vi "Parameter XML Tx - Write old.vi"(0 "String (in)":string, 7 "Database []":T1) -> (4 "String (out)":string)   [LabVIEW 2017]
uses:
  <userlib>/_OpenG.lib/array/array.llb/Remove Duplicates from 1D Array (DBL)__ogtk.vi
  <userlib>/_OpenG.lib/array/array.llb/Filter 1D Array with Scalar (DBL)__ogtk.vi
  <userlib>/_OpenG.lib/array/array.llb/Index 1D Array Elements (DBL)__ogtk.vi
  Controls/Database_Array.ctl
  Controls/Encoding.ctl
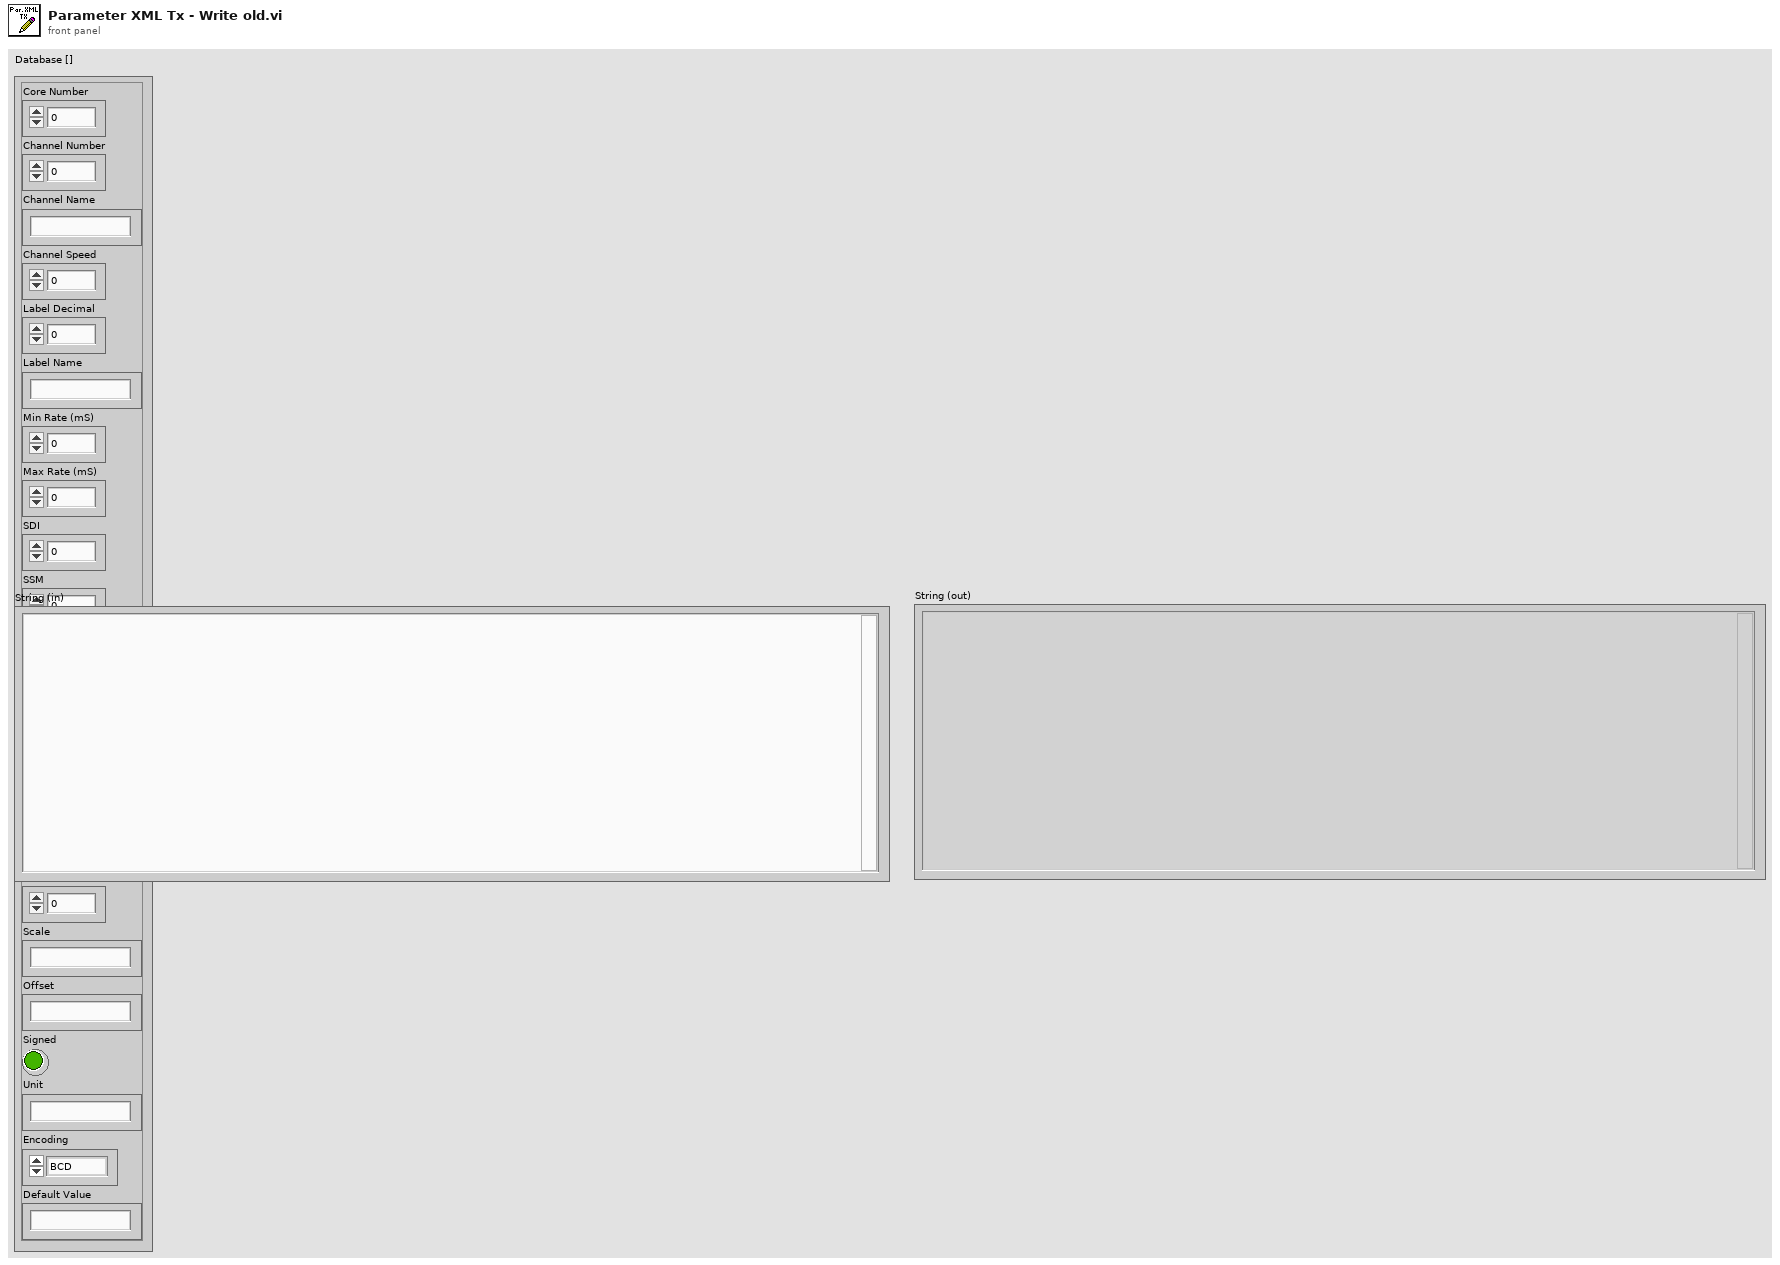
[diagram p1: front panel]
types:
  T1 = typedef "Database_Array.ctl" = cluster{"Core Number":i32, "Channel Number":i32, "Channel Name":string, "Channel Speed":i32, "Label Decimal":i32, "Label Name":string, "Min Rate (mS)":i32, "Max Rate (mS)":i32, "SDI":i32, "SSM":i32, "Create SDI":bool, "Create SSM":bool, "Create Parity":bool, "Parameter Name":string, "Start Bit":i32, "Number of Bits":i32, "Scale":string, "Offset":string, "Signed":bool, "Unit":string, "Encoding":T2, "Default Value":string}
  T2 = typedef "Encoding.ctl" = enum16{"BCD", "BNR", "Discrete"}
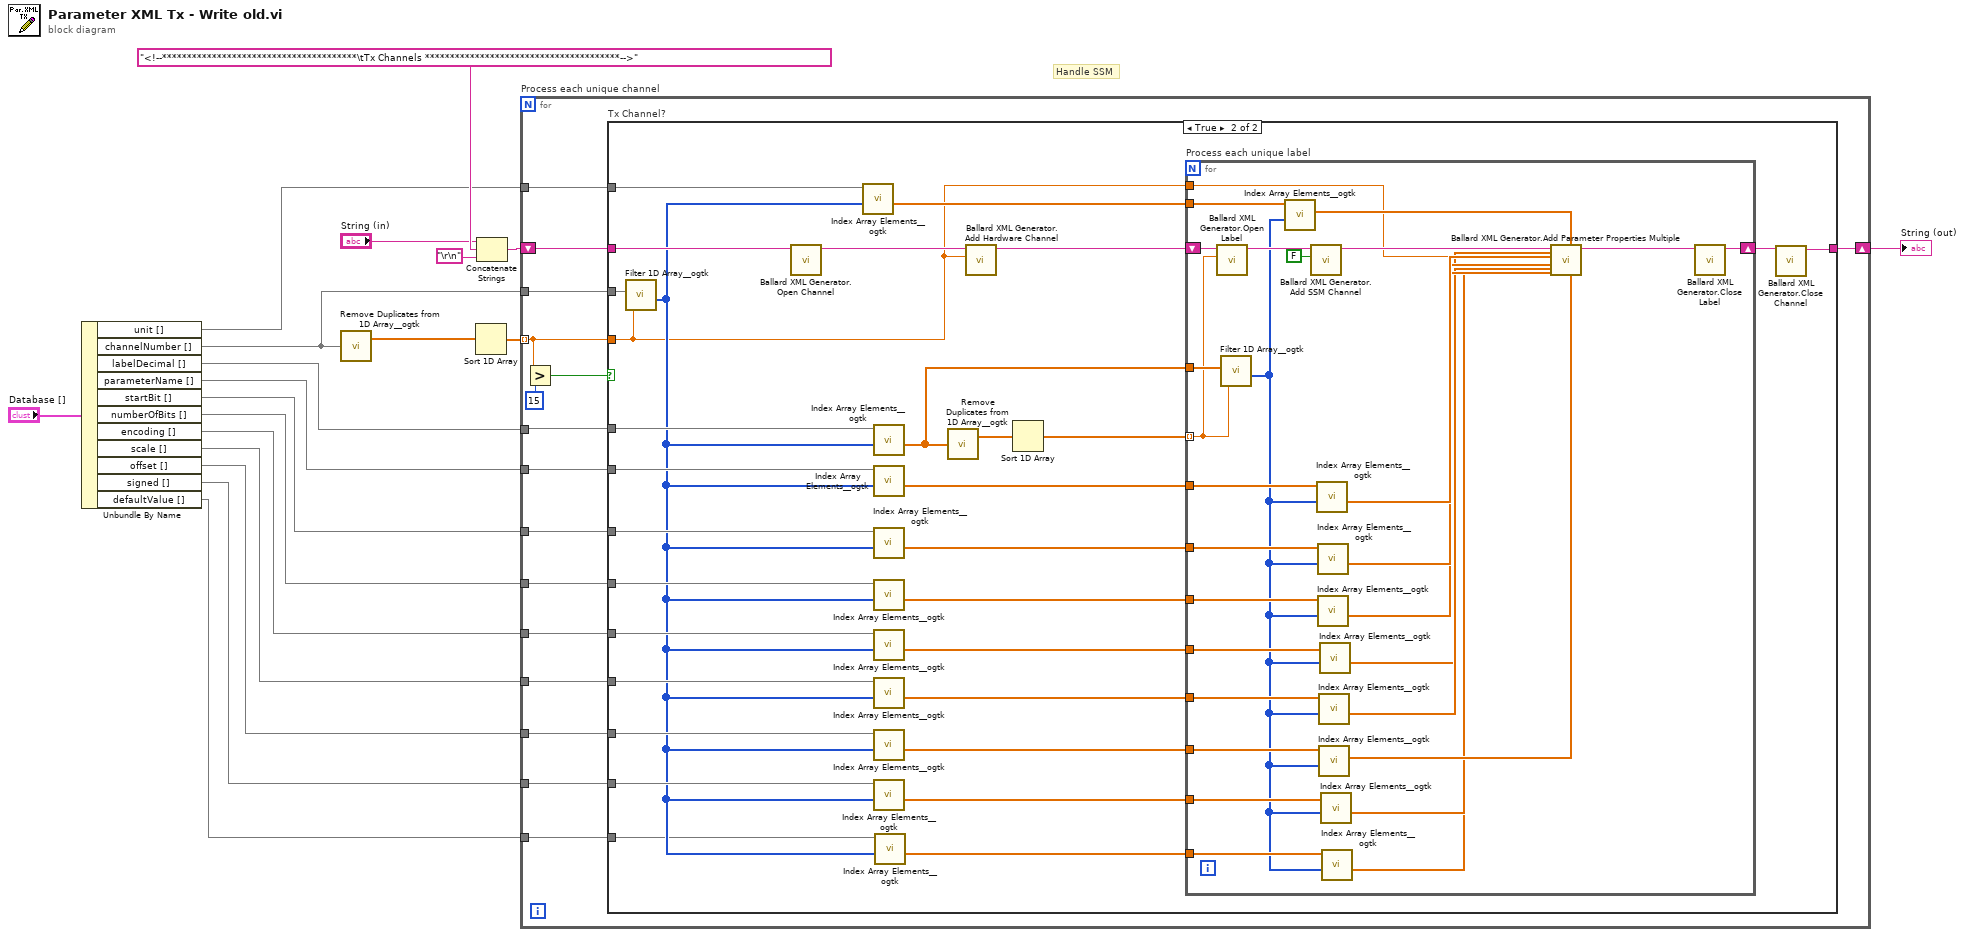
[diagram p0: block diagram]
diagram:
  # "Handle SSM"
  n1 = Unbundle By Name("Database []") -> ("unit []"=w4, "channelNumber []"=w17, "labelDecimal []"=w16, "parameterName []"=w15, "startBit []"=w14, "numberOfBits []"=w9, "encoding []"=w8, "scale []"=w7, "offset []"=w6, "signed []"=w5, "defaultValue []"=w3)
  n2 = call-poly <userlib>:"Remove Duplicates from 1D Array__ogtk.vi"("Input Array"=w17) -> ("Output Array"=w18:dbl[])  [unwired: 1 out]
  n3 = Sort 1D Array(array=w18) -> (sorted array=w19:dbl[])
  n4 = Concatenate Strings("String (in)", "<!--***************************************\tTx Channels ***************************************-->", "\r\n") -> (w10:string)
  n5 = for "Process each unique channel" {
    tunnel: w19 -> [w29] mode=indexing
    tunnel: w17 -> [w35]
    tunnel: w16 -> [w34]
    shift-right: [w32] -> w2
    shift-left: w10 -> [w33]
    tunnel: w15 -> [w31]
    tunnel: w14 -> [w30]
    tunnel: w9 -> [w26]
    tunnel: w8 -> [w25]
    tunnel: w7 -> [w24]
    tunnel: w6 -> [w23]
    tunnel: w5 -> [w22]
    tunnel: w4 -> [w21]
    tunnel: w3 -> [w20]
    n6 = Greater?(x=w29, y=15) -> (0:w28:bool)
    n7 = case "Tx Channel?" shown="True" w28 {
      tunnel: w35 -> [_ w66]
      tunnel: w34 -> [_ w65]
      tunnel: w33 -> [w36 w56]
      tunnel: [w36 w44] -> w32
      tunnel: w31 -> [_ w61]
      tunnel: w30 -> [_ w59]
      tunnel: w29 -> [_ w37]
      tunnel: w26 -> [_ w54]
      tunnel: w25 -> [_ w53]
      tunnel: w24 -> [_ w50]
      tunnel: w23 -> [_ w49]
      tunnel: w22 -> [_ w48]
      tunnel: w21 -> [_ w43]
      tunnel: w20 -> [_ w39]
      frame False {
      }
      frame True {
        n8 = call-poly <userlib>:"Filter 1D Array__ogtk.vi"("items to filter"=w37, "array"=w66) -> ("filtered item indices"=w40:i32[])  [unwired: 4 in, 1 out]
        n9 = call "Ballard XML Generator.Open Channel.vi"("string in"=w56) -> ("string out"=w57:string)  [unwired: 10 in]
        n10 = call-poly <userlib>:"Index Array Elements__ogtk.vi"("indices"=w40, "array"=w43) -> ("elements"=w42:dbl[])  [unwired: 9 in]
        n11 = call-poly <userlib>:"Index Array Elements__ogtk.vi"("indices"=w40, "array"=w65) -> ("elements"=w62:dbl[])  [unwired: 9 in]
        n12 = call-poly <userlib>:"Index Array Elements__ogtk.vi"("indices"=w40, "array"=w61) -> ("elements"=w60:dbl[])  [unwired: 9 in]
        n13 = call-poly <userlib>:"Index Array Elements__ogtk.vi"("indices"=w40, "array"=w59) -> ("elements"=w58:dbl[])  [unwired: 9 in]
        n14 = call-poly <userlib>:"Index Array Elements__ogtk.vi"("indices"=w40, "array"=w54) -> ("elements"=w52:dbl[])  [unwired: 9 in]
        n15 = call-poly <userlib>:"Index Array Elements__ogtk.vi"("indices"=w40, "array"=w53) -> ("elements"=w51:dbl[])  [unwired: 9 in]
        n16 = call-poly <userlib>:"Index Array Elements__ogtk.vi"("indices"=w40, "array"=w50) -> ("elements"=w47:dbl[])  [unwired: 9 in]
        n17 = call-poly <userlib>:"Index Array Elements__ogtk.vi"("indices"=w40, "array"=w49) -> ("elements"=w46:dbl[])  [unwired: 9 in]
        n18 = call-poly <userlib>:"Index Array Elements__ogtk.vi"("indices"=w40, "array"=w48) -> ("elements"=w45:dbl[])  [unwired: 9 in]
        n19 = call-poly <userlib>:"Index Array Elements__ogtk.vi"("indices"=w40, "array"=w39) -> ("elements"=w38:dbl[])  [unwired: 9 in]
        n20 = call-poly <userlib>:"Remove Duplicates from 1D Array__ogtk.vi"("Input Array"=w62) -> ("Output Array"=w64:dbl[])  [unwired: 1 out]
        n21 = call "Ballard XML Generator.Add Hardware Channel.vi"("channel"=w37, "string in"=w57) -> ("string out"=w55:string)  [unwired: 9 in]
        n22 = Sort 1D Array(array=w64) -> (sorted array=w63:dbl[])
        n23 = for "Process each unique label" {
          tunnel: w63 -> [w88] mode=indexing
          tunnel: w62 -> [w94]
          shift-right: [w87] -> w41
          shift-left: w55 -> [w89]
          tunnel: w60 -> [w93]
          tunnel: w58 -> [w92]
          tunnel: w52 -> [w86]
          tunnel: w51 -> [w85]
          tunnel: w47 -> [w84]
          tunnel: w46 -> [w83]
          tunnel: w45 -> [w82]
          tunnel: w42 -> [w81]
          tunnel: w38 -> [w72]
          tunnel: w37 -> [w67]
          n24 = call "Ballard XML Generator.Open Label.vi"("label decimal"=w88, "string in"=w89) -> ("string out"=w91:string)  [unwired: 9 in]
          n25 = call-poly <userlib>:"Filter 1D Array__ogtk.vi"("items to filter"=w88, "array"=w94) -> ("filtered item indices"=w71:i32[])  [unwired: 4 in, 1 out]
          n26 = call-poly <userlib>:"Index Array Elements__ogtk.vi"("indices"=w71, "array"=w81) -> ("elements"=w73:dbl[])  [unwired: 9 in]
          n27 = call "Ballard XML Generator.Add SSM Channel.vi"("create SSM chan?"=FALSE, "string in"=w91) -> ("string out"=w68:string)  [unwired: 9 in]
          n28 = call-poly <userlib>:"Index Array Elements__ogtk.vi"("indices"=w71, "array"=w93) -> ("elements"=w80:dbl[])  [unwired: 9 in]
          n29 = call-poly <userlib>:"Index Array Elements__ogtk.vi"("indices"=w71, "array"=w92) -> ("elements"=w79:dbl[])  [unwired: 9 in]
          n30 = call-poly <userlib>:"Index Array Elements__ogtk.vi"("indices"=w71, "array"=w86) -> ("elements"=w78:dbl[])  [unwired: 9 in]
          n31 = call-poly <userlib>:"Index Array Elements__ogtk.vi"("indices"=w71, "array"=w84) -> ("elements"=w77:dbl[])  [unwired: 9 in]
          n32 = call-poly <userlib>:"Index Array Elements__ogtk.vi"("indices"=w71, "array"=w83) -> ("elements"=w76:dbl[])  [unwired: 9 in]
          n33 = call-poly <userlib>:"Index Array Elements__ogtk.vi"("indices"=w71, "array"=w85) -> ("elements"=w74:dbl[])  [unwired: 9 in]
          n34 = call-poly <userlib>:"Index Array Elements__ogtk.vi"("indices"=w71, "array"=w82) -> ("elements"=w75:dbl[])  [unwired: 9 in]
          n35 = call-poly <userlib>:"Index Array Elements__ogtk.vi"("indices"=w71, "array"=w72) -> ("elements"=w70:dbl[])  [unwired: 9 in]
          n36 = call "Ballard XML Generator.Add Parameter Properties Multiple.vi"(0:w75, 1:w70, 2:w67, 4:w76, 5:w73, 6:w77, "Channel Number"=w74, 8:w78, "Parameter Array"=w79, 10:w80, "string in"=w68) -> ("string out"=w69:string)
          n37 = call "Ballard XML Generator.Close Label.vi"("string in"=w69) -> ("string out"=w87:string)  [unwired: 10 in]
        }
        n38 = call "Ballard XML Generator.Close Channel.vi"("string in"=w41) -> ("string out"=w44:string)  [unwired: 10 in]
      }
    }
  }
  "String (out)" <- w2
